vi "longTime_Queue_task.vi"(8 "error in (no error)":errorcluster, 11 "taskInput":cluster{"State":string, "Parameters":string}) -> (0 "error out":errorcluster, 3 "taskOut":cluster{"State":string, "Parameters":string})   [LabVIEW 2022 SP3]
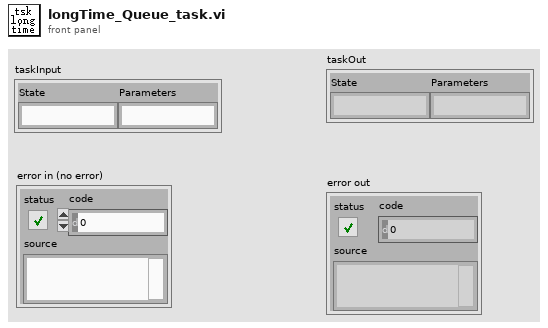
[diagram p1: front panel]
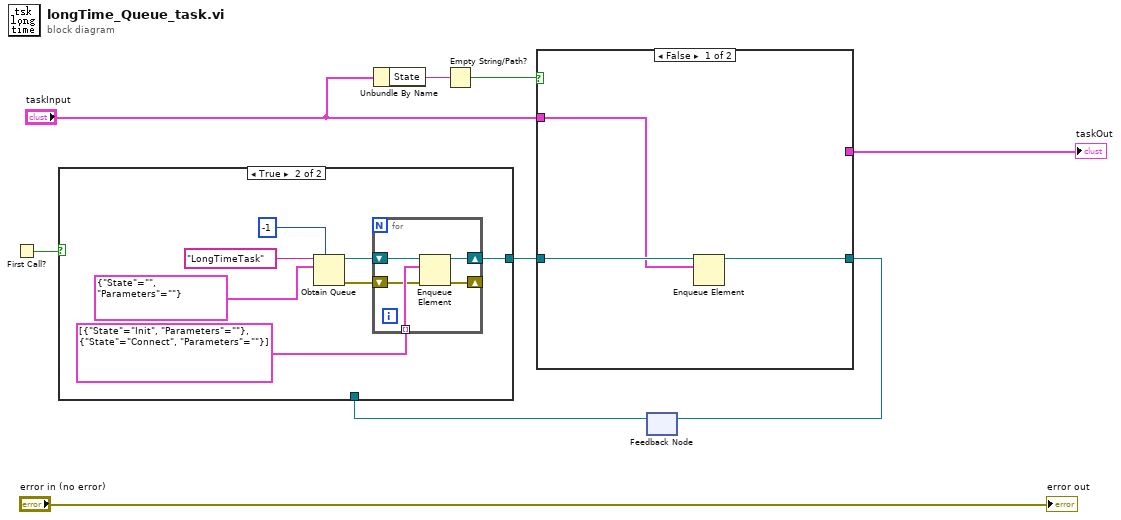
[diagram p0: block diagram]
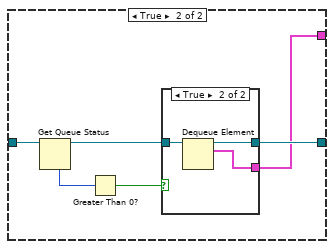
[diagram p2: hidden frame]
diagram:
  n1 = First Call?() -> (First Call?: T/F=w9:bool)
  n2 = Unbundle By Name("taskInput") -> ("State"=w2:string)
  n3 = Empty String/Path?(string/path=w2) -> (empty?=w3:bool)
  n4 = feedback #1() -> (w6:refnum<queue>)  [unwired: 1 in]
  n5 = case shown="True" w9 {
    tunnel: [w10 w14] -> w8
    tunnel: w6 -> [w10 _]
    frame False {
    }
    frame True {
      n6 = Obtain Queue(max queue size (-1, unlimited)=-1, name (unnamed)="LongTimeTask", element data type=cluster{"State":string, "Parameters":string} {"State"="", "Parameters"=""}) -> (queue out=w15:refnum<queue>, error out=w11:errorcluster)  [unwired: 2 in, 1 out]
      n7 = for {
        tunnel: cluster{"State":string, "Parameters":string}[] [{"State"="Init", "Parameters"=""}, {"State"="Connect", "Parameters"=""}] -> [w20] mode=indexing
        shift-right: [w21] -> w14
        shift-left: w15 -> [w22]
        shift-right: [w18] -> _
        shift-left: w11 -> [w19]
        n8 = Enqueue Element(queue=w22, element=w20, error in (no error)=w19) -> (queue out=w21:refnum<queue>, error out=w18:errorcluster)  [unwired: 1 in, 1 out]
      }
    }
  }
  n9 = case shown="False" w3 {
    tunnel: w8 -> [w25 w31]
    tunnel: [w24 w30] -> w7
    tunnel: [_ w27] -> w1
    tunnel: "taskInput" -> [w23 _]
    frame False {
      n10 = Enqueue Element(queue=w25, element=w23) -> (queue out=w24:refnum<queue>)  [unwired: 2 in, 2 out]
    }
    frame True {
      n11 = Get Queue Status(queue=w31) -> (queue out=w29:refnum<queue>, # elements in queue=w28:i32)  [unwired: 2 in, 6 out]
      n12 = Greater Than 0?(x=w28) -> (x > 0?=w26:bool)
      n13 = case shown="True" w26 {
        tunnel: [w32 w35] -> w30
        tunnel: w29 -> [w32 w34]
        tunnel: [_ w33] -> w27
        frame False {
        }
        frame True {
          n14 = Dequeue Element(queue=w34) -> (queue out=w35:refnum<queue>, element=w33:cluster{"State":string, "Parameters":string})  [unwired: 2 in, 2 out]
        }
      }
    }
  }
  "taskOut" <- w1
  n15 = feedback-in #1(w7) -> ()
  "error out" <- "error in (no error)"
